vi "TCam_CenterArray.vi"(0 "Image in":T1, 2 "Point Array":T2[](array[typedef]) {"Y" format="%.2f"; "X" format="%.2f"}, 3 "Size":u32, 5 "draw all?":bool) -> (6 "Image":T1(plugin-control), 7 "Array":cluster{"X":i32, "Y":i32}[][](array[cluster]), 8 "Points":cluster{"X":i32, "Y":i32}[][](array[cluster]))   [LabVIEW 2022 SP3]
uses:
  <vilib>/vision/Image Controls.llb/IMAQ Image.ctl
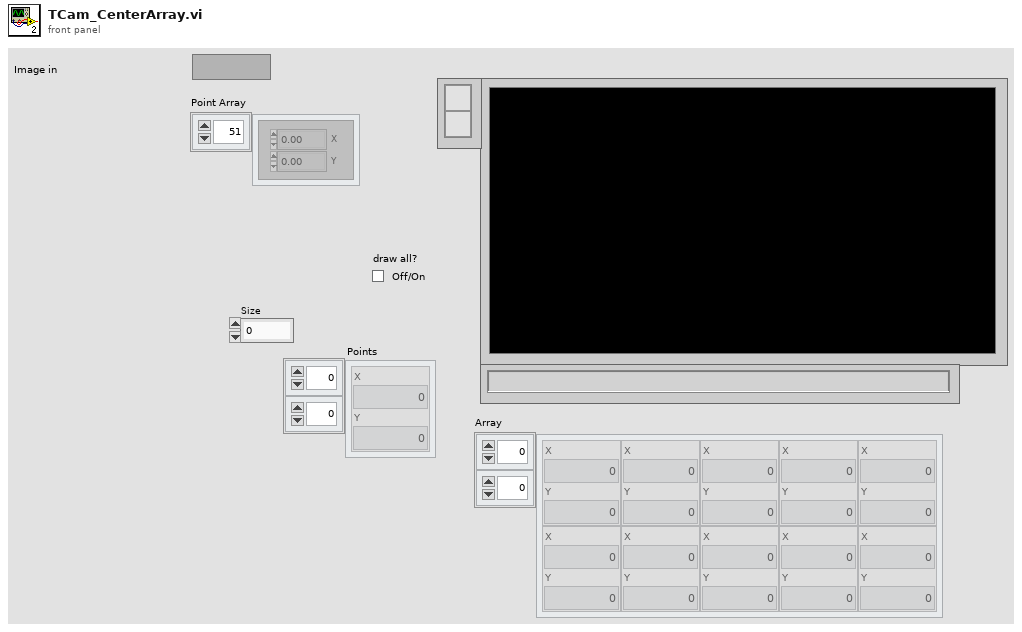
[diagram p1: front panel]
types:
  T1 = typedef "IMAQ Image.ctl" = refnum<image>
  T2 = typedef "IMAQ Point" = cluster{"X":sgl, "Y":sgl}
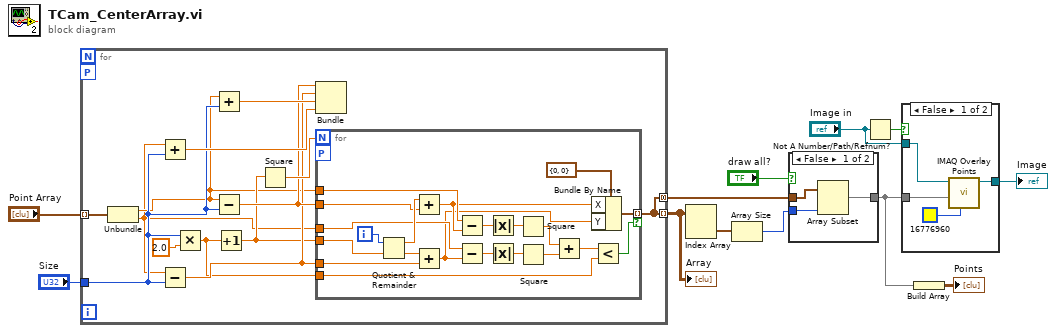
[diagram p0: block diagram]
diagram:
  n1 = for {
    tunnel: "Size" -> [w23]
    tunnel: "Point Array" -> [w18] mode=indexing
    tunnel: [w13] -> w7 mode=indexing
    tunnel: [w13] -> w9 mode=concatenating
    workers-P: _ -> [_]
    n2 = Unbundle(w18) -> ("X"=w16:sgl, "Y"=w15:sgl)
    n3 = Add(x=w15, y=w23) -> (x+y=w24:sgl)
    n4 = Subtract(x=w15, y=w23) -> (x-y=w19:sgl)
    n5 = Multiply(x=w23, y=2.0) -> (x*y=w14:dbl)
    n6 = Add(x=w16, y=w23) -> (x+y=w25:sgl)
    n7 = Subtract(x=w16, y=w23) -> (x-y=w20:sgl)
    n8 = Increment(x=w14) -> (x+1=w17:dbl)
    n9 = Square(x=w17) -> (x^2=w21:dbl)
    n10 = Bundle(w20, w19, w25, w24) -> ()  [unwired: 1 in, 1 out]
    n11 = for {
      N: w21 -> [_]
      tunnel: w17 -> [w45]
      tunnel: w20 -> [w43]
      tunnel: w19 -> [w41]
      tunnel: [w40] -> w13 mode=indexing if=w26
      tunnel: w16 -> [w38]
      tunnel: w15 -> [w31]
      tunnel: w14 -> [w27]
      workers-P: _ -> [_]
      i -> [w46]
      n12 = Quotient & Remainder(x=w46, y=w45) -> (x-y*floor(x/y)=w44:dbl, floor(x/y)=w42:dbl)
      n13 = Add(x=w44, y=w43) -> (x+y=w37:dbl)
      n14 = Add(x=w42, y=w41) -> (x+y=w30:dbl)
      n15 = Subtract(x=w38, y=w37) -> (x-y=w36:dbl)
      n16 = Subtract(x=w31, y=w30) -> (x-y=w33:dbl)
      n17 = Absolute Value(x=w36) -> (abs(x)=w35:dbl)
      n18 = Absolute Value(x=w33) -> (abs(x)=w32:dbl)
      n19 = Square(x=w35) -> (x^2=w34:dbl)
      n20 = Square(x=w32) -> (x^2=w29:dbl)
      n21 = Add(x=w34, y=w29) -> (x+y=w28:dbl)
      n22 = Bundle By Name(cluster=cluster{"X":i32, "Y":i32} {"X"=0, "Y"=0} ("Point"), "X"=w37, "Y"=w30) -> (w40:cluster{"X":i32, "Y":i32})
      n23 = Less?(x=w28, y=w27) -> (x < y?=w26:bool)
    }
  }
  "Array" <- w7
  n24 = Index Array(array=w7) -> (element=w6:cluster{"X":i32, "Y":i32}[])  [unwired: 2 in]
  n25 = Array Size(array=w6) -> (size(s)=w5:i32)
  n26 = case shown="False" "draw all?" {
    tunnel: [w47 w50] -> w2
    tunnel: w9 -> [w49 w50]
    tunnel: w5 -> [w48 _]
    frame False {
      n27 = Array Subset(array=w49, length=w48) -> (w47:cluster{"X":i32, "Y":i32}[])  [unwired: 1 in]
    }
    frame True {
    }
  }
  n28 = Not A Number/Path/Refnum?(number/path/refnum="Image in") -> (NaN/Path/Refnum?=w3:bool)
  n29 = case shown="False" w3 {
    tunnel: [w54 w55] -> w10
    tunnel: w2 -> [w52 _]
    tunnel: "Image in" -> [w51 w55]
    frame False {
      n30 = call "IMAQ Overlay Points"("Color"=u32 16776960, "Array of Points"=w52, "Image"=w51) -> ("Image Out"=w54:T1)  [unwired: 7 in, 1 out]
    }
    frame True {
    }
  }
  "Image" <- w10
  n31 = Build Array(w2) -> (→"Points":cluster{"X":i32, "Y":i32}[][])
